vi "Unit Test.vi"() -> ()   [LabVIEW 2018]
uses:
  BFECC.lvclass
panel:
  in  "Run Chip Image":path
  in  "Save Power Data Path":path
  in  "Start Power Monitor Path":path
  in  "Connect  to FPGA Path":path
  out "error out":errorcluster
  in  "ID or SN":string
  in  "Test File Path":path
  in  "error in (no error)":errorcluster
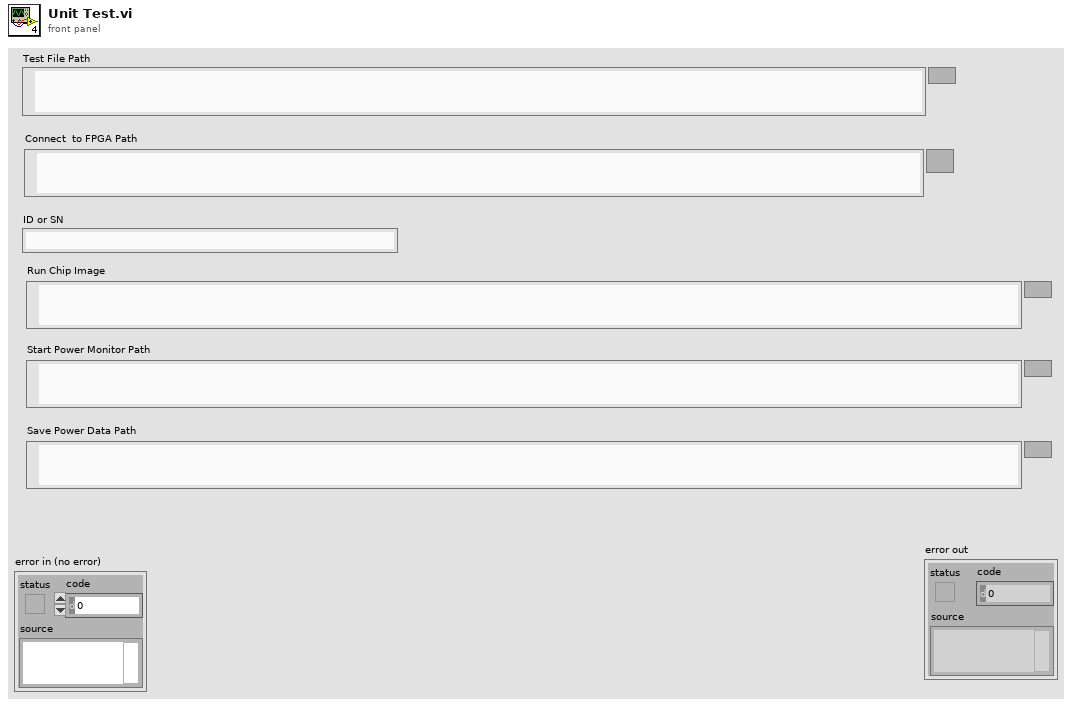
[diagram p1: front panel]
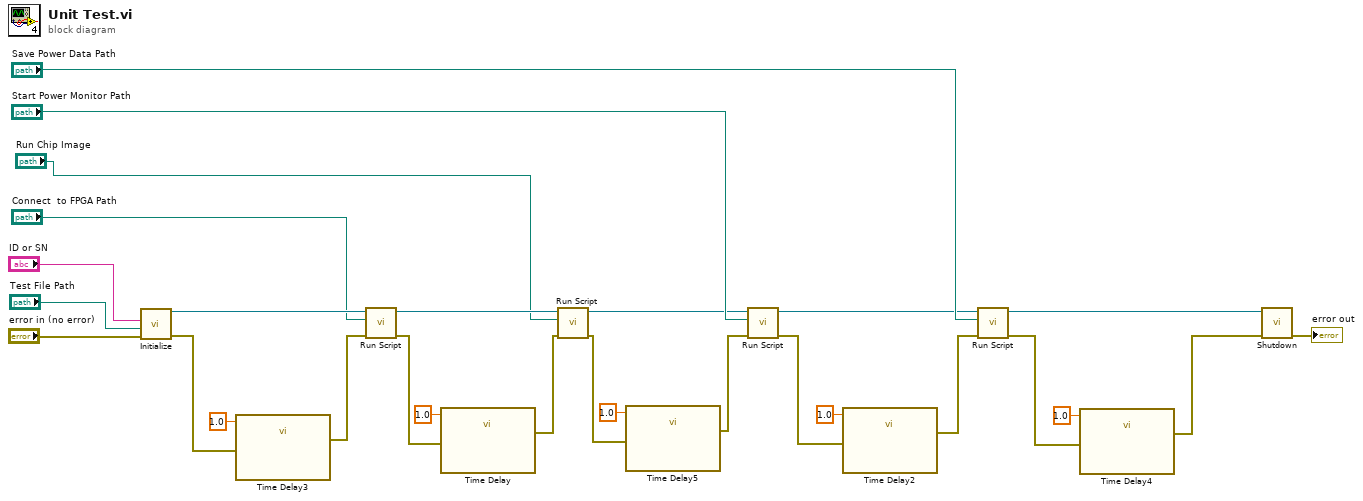
[diagram p0: block diagram]
diagram:
  n1 = call "Initialize.vi"("error in (no error)"="error in (no error)", "Test File Path"="Test File Path", "ID or SN"="ID or SN") -> ("error out"=w19:errorcluster, "BFECC out"=w25:refnum<class "BFECC.lvclass">)  [unwired: 7 in]
  n2 = call "Time Delay3"("error in (no error)"=w19, "Delay Time (s)"=1.0) -> ("error out"=w18:errorcluster)  [unwired: 9 in]
  n3 = call "Run Script.vi"("error in (no error)"=w18, "Script Path"="Connect  to FPGA Path", "BFECC in"=w25) -> ("error out"=w24:errorcluster, "BFECC out"=w4:refnum<class "BFECC.lvclass">)  [unwired: 7 in]
  n4 = call "Time Delay"("error in (no error)"=w24, "Delay Time (s)"=1.0) -> ("error out"=w6:errorcluster)  [unwired: 9 in]
  n5 = call "Run Script.vi"("error in (no error)"=w6, "Script Path"="Run Chip Image", "BFECC in"=w4) -> ("error out"=w5:errorcluster, "BFECC out"=w2:refnum<class "BFECC.lvclass">)  [unwired: 7 in]
  n6 = call "Time Delay5"("error in (no error)"=w5, "Delay Time (s)"=1.0) -> ("error out"=w1:errorcluster)  [unwired: 9 in]
  n7 = call "Run Script.vi"("error in (no error)"=w1, "Script Path"="Start Power Monitor Path", "BFECC in"=w2) -> ("error out"=w15:errorcluster, "BFECC out"=w16:refnum<class "BFECC.lvclass">)  [unwired: 7 in]
  n8 = call "Time Delay2"("error in (no error)"=w15, "Delay Time (s)"=1.0) -> ("error out"=w14:errorcluster)  [unwired: 9 in]
  n9 = call "Run Script.vi"("error in (no error)"=w14, "Script Path"="Save Power Data Path", "BFECC in"=w16) -> ("error out"=w11:errorcluster, "BFECC out"=w10:refnum<class "BFECC.lvclass">)  [unwired: 7 in]
  n10 = call "Time Delay4"("error in (no error)"=w11, "Delay Time (s)"=1.0) -> ("error out"=w9:errorcluster)  [unwired: 9 in]
  n11 = call "Shutdown.vi"("error in (no error)"=w9, "BFECC in"=w10) -> ("error out"=→"error out":errorcluster)  [unwired: 8 in, 1 out]
